vi "MotorControl_PWM+AO.vi"() -> ()   [LabVIEW 2016]
uses:
  <vilib>/Platform/TimedLoop/XDataNode/timing_clust.ctl
  <vilib>/Platform/TimedLoop/XDataNode/nitl_modes.ctl
  <vilib>/Platform/TimedLoop/XDataNode/wakeup.ctl
  <vilib>/rvi/FXPMathLib/FxpDiv/subVIs/nifxpmath_Div_SimConfig.ctl
  <vilib>/rvi/Emulation/niFpgaGetClockAttributes.vi
  <vilib>/rvi/Emulation/niFpgaSctlEmulationGetInTimedLoop.vi
  <vilib>/rvi/Emulation/niFpgaEmulationReportErrorSimple.vi
  <vilib>/rvi/FXPMathLib/FxpDiv/simVIs/DllFxpDivTemp_sub.vi
  GVEncoder.vi
  <vilib>/rvi/Emulation/niFpgaCriticalErrorInLSC.vi
  <vilib>/rvi/Emulation/niFpgaProcessEmulError.vi
  <vilib>/rvi/eio/common/nirviEmuTemplateMethod_errors.vi
  <vilib>/rvi/FXPMathLib/FxpMul/XNode/nifxpmath_Multiplier.xnode
  <vilib>/rvi/FXPMathLib/FxpDiv/XNode/nifxpmath_Div.xnode
  <vilib>/eio/EIONode/EIONode.xnode
  <vilib>/Platform/TimedLoop/XDataNode/XDataNode.xnode
  <vilib>/Platform/TimedLoop/XDataNode/XDNodeRunTimeDep.lvlib
  <vilib>/rvi/FXPMathLib/sim/FxpSim.dll
panel:
  out "ES_PRESSED":bool
  out "PWR_OK":bool
  in  "PWM (Hz/A)":fxp<+/-,32,16>=13.333328247070312 format="%#_21g"
  in  "EncdRst":bool[](array[boolean])=[FALSE, FALSE, FALSE, FALSE, FALSE, FALSE, FALSE, FALSE]
  out "PWM":fxp<+,16,8>[](array[numeric])
  in  "AmpCmd":sgl[](array[numeric])=[0.0, 0.0, 0.0, 0.0, 0.0, 0.0, 0.0, 0.0] format="%#.3f"
  in  "DisableWhenNotReady":bool
  in  "EnableMaster":bool
  out "Ready":bool[](array[boolean])
  in  "Enable":bool[](array[boolean])=[FALSE, FALSE, FALSE, FALSE, FALSE, FALSE, FALSE, FALSE]
  in  "EncoderCount":fxp<+,16,16>=500.0
  in  "2pi":fxp<+/-,32,10>=6.283185243606567 format="%#_39g"
  out "EncdAngle":sgl[](array[numeric]) format="%#.3f"
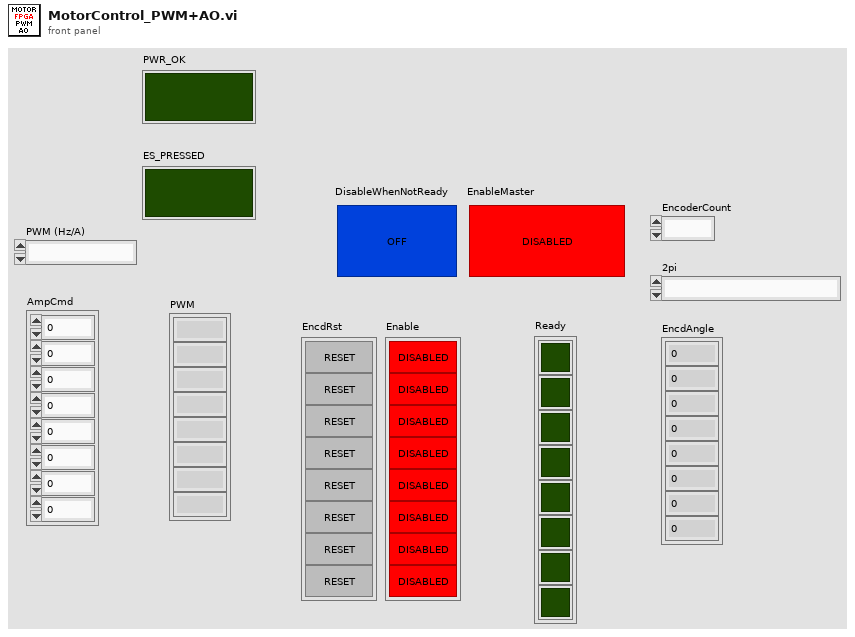
[diagram p1: front panel]
types:
  T1 = typedef "XDNodeRunTimeDep.lvlib/timing_clust.ctl" = cluster{"Expected End [f-1]":u64, "Actual End [f-1]":u64, "Finished Late? [f-1]":bool, "Expected End [i-1]":u64, "Actual End [i-1]":u64, "Finished Late? [i-1]":bool, "Expected Start [i]":u64, "Actual Start [i]":u64, "Expected Start [f]":u64, "Actual Start [f]":u64, "Source Name":string, "Structure Name":string, "Period":i64, "Deadline":i64, "Offset":i64, "Start":i64, "Priority":i32, "Timeout":i32, "Mode":T2, "Wakeup Reason":T3, "Error":errorcluster, "Source Type":string, "Secondary Source Type":string, "Global End Time":u64, "Global Start Time":u64, "Frame Duration":u64, "Iteration Duration":u64, "Assigned CPU":i32, "I/O Scan Engine Mode":u32}
  T2 = typedef "XDNodeRunTimeDep.lvlib/nitl_modes.ctl" = enum32{"No Change", "Process missed periods, maintain original phase", "Discard missed periods, maintain original phase", "Process missed periods, ignore original phase", "Discard missed periods, ignore original phase"}
  T3 = typedef "XDNodeRunTimeDep.lvlib/wakeup.ctl" = enum32{"Normal", "Aborted", "Asynchronous wakeup", "Timing source error", "Timed loop error", "Timeout"}
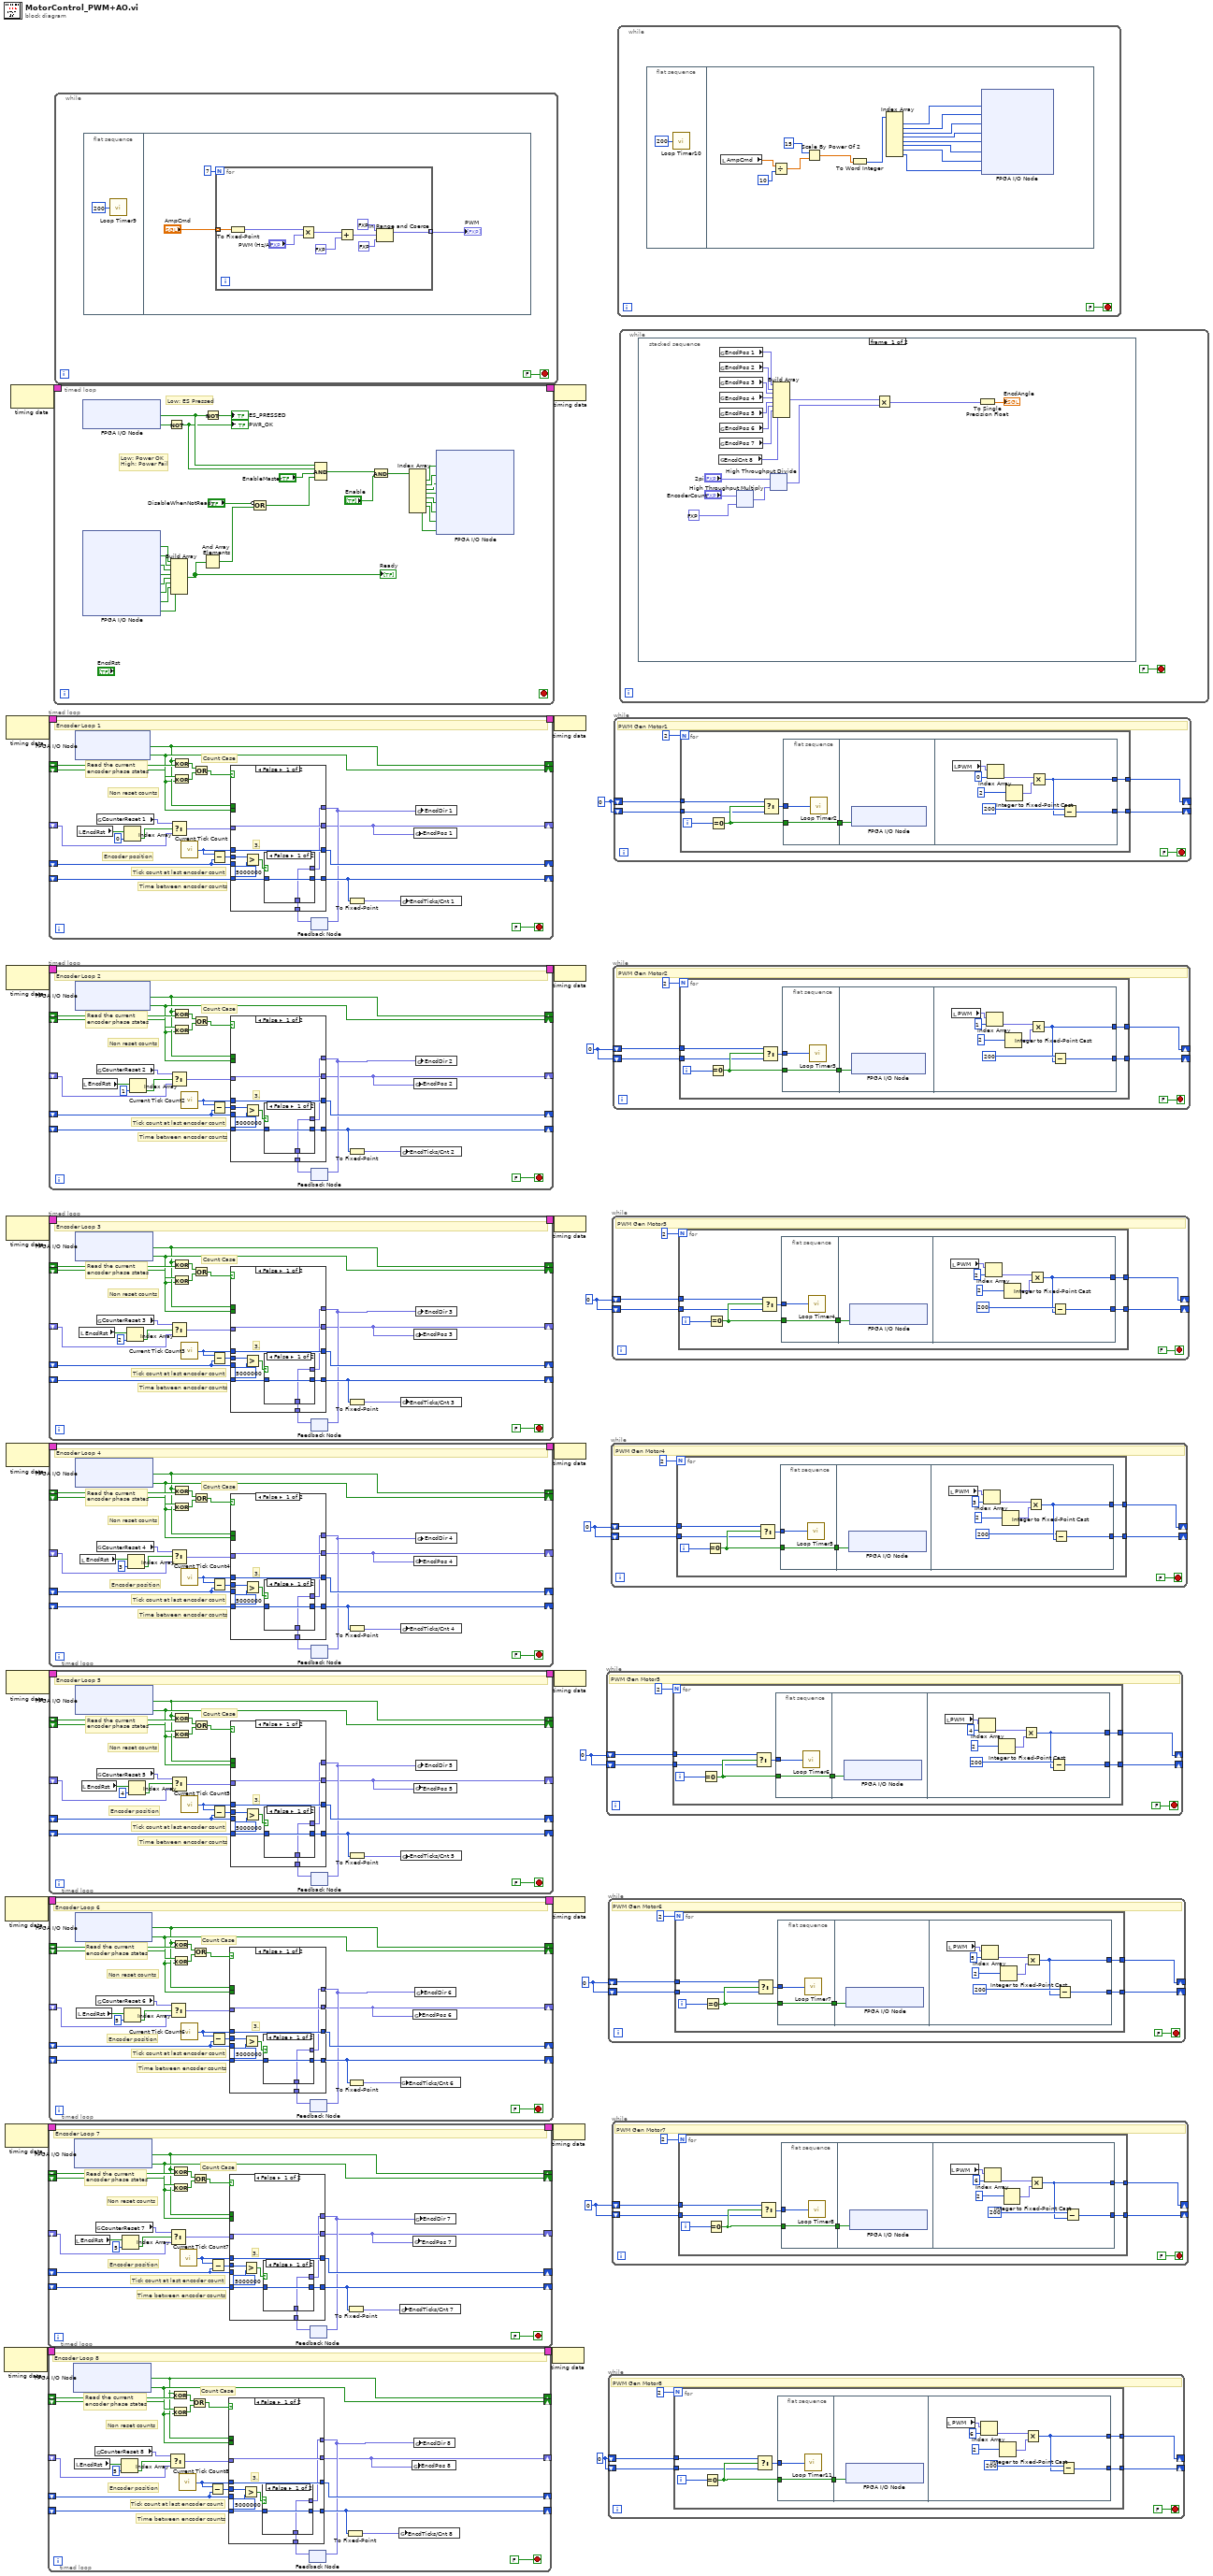
[diagram p0: block diagram]
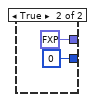
[diagram p2: hidden frame]
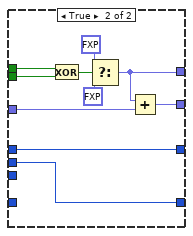
[diagram p3: hidden frame]
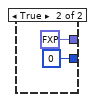
[diagram p4: hidden frame]
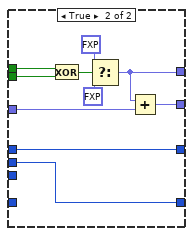
[diagram p5: hidden frame]
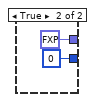
[diagram p6: hidden frame]
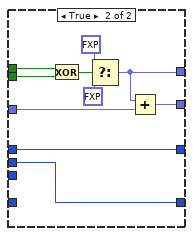
[diagram p7: hidden frame]
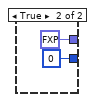
[diagram p8: hidden frame]
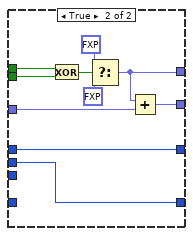
[diagram p9: hidden frame]
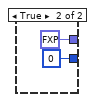
[diagram p10: hidden frame]
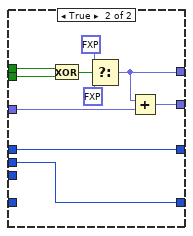
[diagram p11: hidden frame]
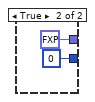
[diagram p12: hidden frame]
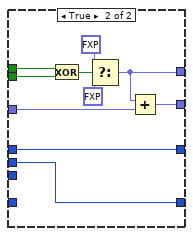
[diagram p13: hidden frame]
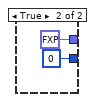
[diagram p14: hidden frame]
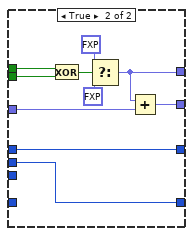
[diagram p15: hidden frame]
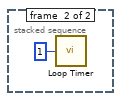
[diagram p16: hidden frame]
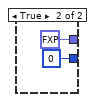
[diagram p17: hidden frame]
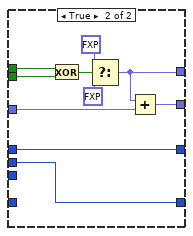
[diagram p18: hidden frame]
diagram:
  w1 = u32 0
  w4 = u32 0
  w5 = u32 0
  w6 = u32 0
  w7 = u32 0
  w8 = u32 0
  w9 = u32 0
  w10 = u32 0
  n1 = node-c288() -> (w3:T1)  [unwired: 1 in]
  n2 = node-c288() -> (w14:T1)  [unwired: 1 in]
  n3 = node-c288() -> (w16:T1)  [unwired: 1 in]
  n4 = node-c288() -> (w26:T1)  [unwired: 1 in]
  n5 = node-c288() -> (w24:T1)  [unwired: 1 in]
  n6 = node-c288() -> (w22:T1)  [unwired: 1 in]
  n7 = node-c288() -> (w20:T1)  [unwired: 1 in]
  n8 = node-c288() -> (w18:T1)  [unwired: 1 in]
  n9 = node-c288() -> (w12:T1)  [unwired: 1 in]
  n10 = timed-loop {
    shift-right: [w44] -> _
    shift-left: _ -> [w50]
    shift-right: [w45] -> _
    shift-left: _ -> [w43]
    shift-right: [w31] -> _
    shift-left: _ -> [w49]
    shift-right: [w48] -> _
    shift-left: _ -> [w42]
    shift-right: [w35] -> _
    shift-left: _ -> [w47]
    timing: w3 -> [_]
    timing-out: [_] -> w2
    stop <- FALSE stop-if-true
    # "Count Case"
    # "Read the current\nencoder phase states"
    # "Non reset counts"
    # "Encoder position"
    # "Time between encoder counts"
    # "Tick count at last encoder count"
    # "Encoder Loop 8"
    n11 = xnode "FPGA I/O Node"() -> ("Connector1/DIO38"=w44:bool, "Connector1/DIO39"=w45:bool)  [unwired: 2 in, 2 out]
    n12 = local read "EncdRst"() -> (w29:bool[])
    n13 = global read "GVEncoder.vi" "CounterReset 8"() -> (w32:fxp<+/-,32,32>)
    n14 = Index Array(array=w29, index=5) -> (element=w27:bool)
    n15 = Select(t=w32, s=w27, f=w49) -> (s? t:f=w38:fxp<+/-,32,32>)
    n16 = Exclusive Or(1:w50, 2:w44) -> (0:w41:bool)
    n17 = Exclusive Or(1:w43, 2:w45) -> (0:w40:bool)
    n18 = call "Current Tick Count8"() -> ("Tick Count(Ticks)"=w36:u32)
    n19 = Or(x=w41, y=w40) -> (x .or. y?=w39:bool)
    n20 = Subtract(x=w36, y=w42) -> (x-y=w37:u32)
    n21 = feedback #1() -> (w34:fxp<+/-,2,2>)  [unwired: 1 in]
    n22 = case shown="False" w39 {
      tunnel: [w59 w67] -> w31
      tunnel: w38 -> [w59 w73]
      tunnel: [w53 w66] -> w48
      tunnel: w42 -> [w53 _]
      tunnel: [w56 w65] -> w35
      tunnel: w47 -> [w55 _]
      tunnel: w44 -> [_ w69]
      tunnel: w43 -> [_ w68]
      tunnel: w37 -> [w54 w65]
      tunnel: w36 -> [_ w66]
      tunnel: [w52 w64] -> w33
      tunnel: w34 -> [w51 _]
      frame False {
        # "3."
        n23 = Greater?(x=w54, y=u32 5000000 ("x")) -> (0:w57:bool)
        n24 = case shown="False" w57 {
          tunnel: [w61 u32 0 ("x")] -> w56
          tunnel: w55 -> [w61 _]
          tunnel: [w60 fxp<+/-,2,2> 0.0 ("16 bit")] -> w52
          tunnel: w51 -> [w60 _]
          frame False {
          }
          frame True {
          }
        }
      }
      frame True {
        n25 = Exclusive Or(1:w68, 2:w69) -> (0:w70:bool)
        n26 = Select(t=fxp<+,1,1> 1.0 ("16 bit"), s=w70, f=fxp<+/-,1,1> -1.0 ("16 bit")) -> (s? t:f=w64:fxp<+/-,2,2>)
        n27 = Add(x=w64, y=w73) -> (x+y=w67:fxp<+/-,32,32>)
      }
    }
    n28 = feedback-in #1(w33) -> ()
    n29 = To Fixed-Point(number=w35) -> (fixed-point=w30:fxp<+,32,32>)  [unwired: 1 in]
    n30 = global write "GVEncoder.vi" "EncdTicks/Cnt 8"(w30) -> ()
    n31 = global write "GVEncoder.vi" "EncdPos 8"(w31) -> ()
    n32 = global write "GVEncoder.vi" "EncdDir 8"(w33) -> ()
  }
  n33 = timed-loop {
    shift-right: [w93] -> _
    shift-left: _ -> [w99]
    shift-right: [w94] -> _
    shift-left: _ -> [w92]
    shift-right: [w80] -> _
    shift-left: _ -> [w98]
    shift-right: [w97] -> _
    shift-left: _ -> [w91]
    shift-right: [w84] -> _
    shift-left: _ -> [w96]
    timing: w14 -> [_]
    timing-out: [_] -> w13
    stop <- FALSE stop-if-true
    # "Count Case"
    # "Read the current\nencoder phase states"
    # "Non reset counts"
    # "Encoder position"
    # "Time between encoder counts"
    # "Tick count at last encoder count"
    # "Encoder Loop 7"
    n34 = xnode "FPGA I/O Node"() -> ("Connector1/DIO33"=w93:bool, "Connector1/DIO34"=w94:bool)  [unwired: 2 in, 2 out]
    n35 = local read "EncdRst"() -> (w78:bool[])
    n36 = global read "GVEncoder.vi" "CounterReset 7"() -> (w81:fxp<+/-,32,32>)
    n37 = Index Array(array=w78, index=5) -> (element=w76:bool)
    n38 = Select(t=w81, s=w76, f=w98) -> (s? t:f=w87:fxp<+/-,32,32>)
    n39 = Exclusive Or(1:w99, 2:w93) -> (0:w90:bool)
    n40 = Exclusive Or(1:w92, 2:w94) -> (0:w89:bool)
    n41 = call "Current Tick Count7"() -> ("Tick Count(Ticks)"=w85:u32)
    n42 = Or(x=w90, y=w89) -> (x .or. y?=w88:bool)
    n43 = Subtract(x=w85, y=w91) -> (x-y=w86:u32)
    n44 = feedback #2() -> (w83:fxp<+/-,2,2>)  [unwired: 1 in]
    n45 = case shown="False" w88 {
      tunnel: [w108 w116] -> w80
      tunnel: w87 -> [w108 w122]
      tunnel: [w102 w115] -> w97
      tunnel: w91 -> [w102 _]
      tunnel: [w105 w114] -> w84
      tunnel: w96 -> [w104 _]
      tunnel: w93 -> [_ w118]
      tunnel: w92 -> [_ w117]
      tunnel: w86 -> [w103 w114]
      tunnel: w85 -> [_ w115]
      tunnel: [w101 w113] -> w82
      tunnel: w83 -> [w100 _]
      frame False {
        # "3."
        n46 = Greater?(x=w103, y=u32 5000000 ("x")) -> (0:w106:bool)
        n47 = case shown="False" w106 {
          tunnel: [w110 u32 0 ("x")] -> w105
          tunnel: w104 -> [w110 _]
          tunnel: [w109 fxp<+/-,2,2> 0.0 ("16 bit")] -> w101
          tunnel: w100 -> [w109 _]
          frame False {
          }
          frame True {
          }
        }
      }
      frame True {
        n48 = Exclusive Or(1:w117, 2:w118) -> (0:w119:bool)
        n49 = Select(t=fxp<+,1,1> 1.0 ("16 bit"), s=w119, f=fxp<+/-,1,1> -1.0 ("16 bit")) -> (s? t:f=w113:fxp<+/-,2,2>)
        n50 = Add(x=w113, y=w122) -> (x+y=w116:fxp<+/-,32,32>)
      }
    }
    n51 = feedback-in #2(w82) -> ()
    n52 = To Fixed-Point(number=w84) -> (fixed-point=w79:fxp<+,32,32>)  [unwired: 1 in]
    n53 = global write "GVEncoder.vi" "EncdTicks/Cnt 7"(w79) -> ()
    n54 = global write "GVEncoder.vi" "EncdPos 7"(w80) -> ()
    n55 = global write "GVEncoder.vi" "EncdDir 7"(w82) -> ()
  }
  n56 = timed-loop {
    shift-right: [w142] -> _
    shift-left: _ -> [w148]
    shift-right: [w143] -> _
    shift-left: _ -> [w141]
    shift-right: [w129] -> _
    shift-left: _ -> [w147]
    shift-right: [w146] -> _
    shift-left: _ -> [w140]
    shift-right: [w133] -> _
    shift-left: _ -> [w145]
    timing: w16 -> [_]
    timing-out: [_] -> w15
    stop <- FALSE stop-if-true
    # "Count Case"
    # "Read the current\nencoder phase states"
    # "Non reset counts"
    # "Encoder position"
    # "Time between encoder counts"
    # "Tick count at last encoder count"
    # "Encoder Loop 6"
    n57 = xnode "FPGA I/O Node"() -> ("Connector1/DIO28"=w142:bool, "Connector1/DIO29"=w143:bool)  [unwired: 2 in, 2 out]
    n58 = local read "EncdRst"() -> (w126:bool[])
    n59 = global read "GVEncoder.vi" "CounterReset 6"() -> (w130:fxp<+/-,32,32>)
    n60 = Index Array(array=w126, index=5) -> (element=w125:bool)
    n61 = Select(t=w130, s=w125, f=w147) -> (s? t:f=w136:fxp<+/-,32,32>)
    n62 = Exclusive Or(1:w148, 2:w142) -> (0:w139:bool)
    n63 = Exclusive Or(1:w141, 2:w143) -> (0:w138:bool)
    n64 = call "Current Tick Count6"() -> ("Tick Count(Ticks)"=w134:u32)
    n65 = Or(x=w139, y=w138) -> (x .or. y?=w137:bool)
    n66 = Subtract(x=w134, y=w140) -> (x-y=w135:u32)
    n67 = feedback #3() -> (w132:fxp<+/-,2,2>)  [unwired: 1 in]
    n68 = case shown="False" w137 {
      tunnel: [w157 w165] -> w129
      tunnel: w136 -> [w157 w171]
      tunnel: [w151 w164] -> w146
      tunnel: w140 -> [w151 _]
      tunnel: [w154 w163] -> w133
      tunnel: w145 -> [w153 _]
      tunnel: w142 -> [_ w167]
      tunnel: w141 -> [_ w166]
      tunnel: w135 -> [w152 w163]
      tunnel: w134 -> [_ w164]
      tunnel: [w150 w162] -> w131
      tunnel: w132 -> [w149 _]
      frame False {
        # "3."
        n69 = Greater?(x=w152, y=u32 5000000 ("x")) -> (0:w155:bool)
        n70 = case shown="False" w155 {
          tunnel: [w159 u32 0 ("x")] -> w154
          tunnel: w153 -> [w159 _]
          tunnel: [w158 fxp<+/-,2,2> 0.0 ("16 bit")] -> w150
          tunnel: w149 -> [w158 _]
          frame False {
          }
          frame True {
          }
        }
      }
      frame True {
        n71 = Exclusive Or(1:w166, 2:w167) -> (0:w168:bool)
        n72 = Select(t=fxp<+,1,1> 1.0 ("16 bit"), s=w168, f=fxp<+/-,1,1> -1.0 ("16 bit")) -> (s? t:f=w162:fxp<+/-,2,2>)
        n73 = Add(x=w162, y=w171) -> (x+y=w165:fxp<+/-,32,32>)
      }
    }
    n74 = feedback-in #3(w131) -> ()
    n75 = To Fixed-Point(number=w133) -> (fixed-point=w128:fxp<+,32,32>)  [unwired: 1 in]
    n76 = global write "GVEncoder.vi" "EncdTicks/Cnt 6"(w128) -> ()
    n77 = global write "GVEncoder.vi" "EncdPos 6"(w129) -> ()
    n78 = global write "GVEncoder.vi" "EncdDir 6"(w131) -> ()
  }
  n79 = timed-loop {
    shift-right: [w191] -> _
    shift-left: _ -> [w197]
    shift-right: [w192] -> _
    shift-left: _ -> [w190]
    shift-right: [w178] -> _
    shift-left: _ -> [w196]
    shift-right: [w195] -> _
    shift-left: _ -> [w189]
    shift-right: [w182] -> _
    shift-left: _ -> [w194]
    timing: w26 -> [_]
    timing-out: [_] -> w25
    stop <- FALSE stop-if-true
    # "Count Case"
    # "Read the current\nencoder phase states"
    # "Non reset counts"
    # "Encoder position"
    # "Time between encoder counts"
    # "Tick count at last encoder count"
    # "Encoder Loop 1"
    n80 = xnode "FPGA I/O Node"() -> ("Connector1/DIO3"=w191:bool, "Connector1/DIO4"=w192:bool)  [unwired: 2 in, 2 out]
    n81 = local read "EncdRst"() -> (w176:bool[])
    n82 = global read "GVEncoder.vi" "CounterReset 1"() -> (w179:fxp<+/-,32,32>)
    n83 = Index Array(array=w176, index=0) -> (element=w174:bool)
    n84 = Select(t=w179, s=w174, f=w196) -> (s? t:f=w185:fxp<+/-,32,32>)
    n85 = Exclusive Or(1:w197, 2:w191) -> (0:w188:bool)
    n86 = Exclusive Or(1:w190, 2:w192) -> (0:w187:bool)
    n87 = call "Current Tick Count"() -> ("Tick Count(Ticks)"=w183:u32)
    n88 = Or(x=w188, y=w187) -> (x .or. y?=w186:bool)
    n89 = Subtract(x=w183, y=w189) -> (x-y=w184:u32)
    n90 = feedback #4() -> (w181:fxp<+/-,2,2>)  [unwired: 1 in]
    n91 = case shown="False" w186 {
      tunnel: [w206 w214] -> w178
      tunnel: w185 -> [w206 w220]
      tunnel: [w200 w213] -> w195
      tunnel: w189 -> [w200 _]
      tunnel: [w203 w212] -> w182
      tunnel: w194 -> [w202 _]
      tunnel: w191 -> [_ w216]
      tunnel: w190 -> [_ w215]
      tunnel: w184 -> [w201 w212]
      tunnel: w183 -> [_ w213]
      tunnel: [w199 w211] -> w180
      tunnel: w181 -> [w198 _]
      frame False {
        # "3."
        n92 = Greater?(x=w201, y=u32 5000000 ("x")) -> (0:w204:bool)
        n93 = case shown="False" w204 {
          tunnel: [w208 u32 0 ("x")] -> w203
          tunnel: w202 -> [w208 _]
          tunnel: [w207 fxp<+/-,2,2> 0.0 ("16 bit")] -> w199
          tunnel: w198 -> [w207 _]
          frame False {
          }
          frame True {
          }
        }
      }
      frame True {
        n94 = Exclusive Or(1:w215, 2:w216) -> (0:w217:bool)
        n95 = Select(t=fxp<+,1,1> 1.0 ("16 bit"), s=w217, f=fxp<+/-,1,1> -1.0 ("16 bit")) -> (s? t:f=w211:fxp<+/-,2,2>)
        n96 = Add(x=w211, y=w220) -> (x+y=w214:fxp<+/-,32,32>)
      }
    }
    n97 = feedback-in #4(w180) -> ()
    n98 = To Fixed-Point(number=w182) -> (fixed-point=w177:fxp<+,32,32>)  [unwired: 1 in]
    n99 = global write "GVEncoder.vi" "EncdTicks/Cnt 1"(w177) -> ()
    n100 = global write "GVEncoder.vi" "EncdPos 1"(w178) -> ()
    n101 = global write "GVEncoder.vi" "EncdDir 1"(w180) -> ()
  }
  n102 = timed-loop {
    shift-right: [w240] -> _
    shift-left: _ -> [w246]
    shift-right: [w241] -> _
    shift-left: _ -> [w239]
    shift-right: [w227] -> _
    shift-left: _ -> [w245]
    shift-right: [w244] -> _
    shift-left: _ -> [w238]
    shift-right: [w231] -> _
    shift-left: _ -> [w243]
    timing: w24 -> [_]
    timing-out: [_] -> w23
    stop <- FALSE stop-if-true
    # "Count Case"
    # "Read the current\nencoder phase states"
    # "Non reset counts"
    # "Time between encoder counts"
    # "Tick count at last encoder count"
    # "Encoder Loop 2"
    n103 = xnode "FPGA I/O Node"() -> ("Connector1/DIO8"=w240:bool, "Connector1/DIO9"=w241:bool)  [unwired: 2 in, 2 out]
    n104 = local read "EncdRst"() -> (w224:bool[])
    n105 = global read "GVEncoder.vi" "CounterReset 2"() -> (w228:fxp<+/-,32,32>)
    n106 = Index Array(array=w224, index=1) -> (element=w223:bool)
    n107 = Select(t=w228, s=w223, f=w245) -> (s? t:f=w234:fxp<+/-,32,32>)
    n108 = Exclusive Or(1:w246, 2:w240) -> (0:w237:bool)
    n109 = Exclusive Or(1:w239, 2:w241) -> (0:w236:bool)
    n110 = call "Current Tick Count2"() -> ("Tick Count(Ticks)"=w232:u32)
    n111 = Or(x=w237, y=w236) -> (x .or. y?=w235:bool)
    n112 = Subtract(x=w232, y=w238) -> (x-y=w233:u32)
    n113 = feedback #5() -> (w230:fxp<+/-,2,2>)  [unwired: 1 in]
    n114 = case shown="False" w235 {
      tunnel: [w255 w263] -> w227
      tunnel: w234 -> [w255 w269]
      tunnel: [w249 w262] -> w244
      tunnel: w238 -> [w249 _]
      tunnel: [w252 w261] -> w231
      tunnel: w243 -> [w251 _]
      tunnel: w240 -> [_ w265]
      tunnel: w239 -> [_ w264]
      tunnel: w233 -> [w250 w261]
      tunnel: w232 -> [_ w262]
      tunnel: [w248 w260] -> w229
      tunnel: w230 -> [w247 _]
      frame False {
        # "3."
        n115 = Greater?(x=w250, y=u32 5000000 ("x")) -> (0:w253:bool)
        n116 = case shown="False" w253 {
          tunnel: [w257 u32 0 ("x")] -> w252
          tunnel: w251 -> [w257 _]
          tunnel: [w256 fxp<+/-,2,2> 0.0 ("16 bit")] -> w248
          tunnel: w247 -> [w256 _]
          frame False {
          }
          frame True {
          }
        }
      }
      frame True {
        n117 = Exclusive Or(1:w264, 2:w265) -> (0:w266:bool)
        n118 = Select(t=fxp<+,1,1> 1.0 ("16 bit"), s=w266, f=fxp<+/-,1,1> -1.0 ("16 bit")) -> (s? t:f=w260:fxp<+/-,2,2>)
        n119 = Add(x=w260, y=w269) -> (x+y=w263:fxp<+/-,32,32>)
      }
    }
    n120 = feedback-in #5(w229) -> ()
    n121 = To Fixed-Point(number=w231) -> (fixed-point=w226:fxp<+,32,32>)  [unwired: 1 in]
    n122 = global write "GVEncoder.vi" "EncdTicks/Cnt 2"(w226) -> ()
    n123 = global write "GVEncoder.vi" "EncdPos 2"(w227) -> ()
    n124 = global write "GVEncoder.vi" "EncdDir 2"(w229) -> ()
  }
  n125 = timed-loop {
    shift-right: [w289] -> _
    shift-left: _ -> [w295]
    shift-right: [w290] -> _
    shift-left: _ -> [w288]
    shift-right: [w276] -> _
    shift-left: _ -> [w294]
    shift-right: [w293] -> _
    shift-left: _ -> [w287]
    shift-right: [w280] -> _
    shift-left: _ -> [w292]
    timing: w22 -> [_]
    timing-out: [_] -> w21
    stop <- FALSE stop-if-true
    # "Count Case"
    # "Read the current\nencoder phase states"
    # "Non reset counts"
    # "Time between encoder counts"
    # "Tick count at last encoder count"
    # "Encoder Loop 3"
    n126 = xnode "FPGA I/O Node"() -> ("Connector1/DIO13"=w289:bool, "Connector1/DIO14"=w290:bool)  [unwired: 2 in, 2 out]
    n127 = local read "EncdRst"() -> (w274:bool[])
    n128 = global read "GVEncoder.vi" "CounterReset 3"() -> (w277:fxp<+/-,32,32>)
    n129 = Index Array(array=w274, index=2) -> (element=w272:bool)
    n130 = Select(t=w277, s=w272, f=w294) -> (s? t:f=w283:fxp<+/-,32,32>)
    n131 = Exclusive Or(1:w295, 2:w289) -> (0:w286:bool)
    n132 = Exclusive Or(1:w288, 2:w290) -> (0:w285:bool)
    n133 = call "Current Tick Count3"() -> ("Tick Count(Ticks)"=w281:u32)
    n134 = Or(x=w286, y=w285) -> (x .or. y?=w284:bool)
    n135 = Subtract(x=w281, y=w287) -> (x-y=w282:u32)
    n136 = feedback #6() -> (w279:fxp<+/-,2,2>)  [unwired: 1 in]
    n137 = case shown="False" w284 {
      tunnel: [w304 w312] -> w276
      tunnel: w283 -> [w304 w318]
      tunnel: [w298 w311] -> w293
      tunnel: w287 -> [w298 _]
      tunnel: [w301 w310] -> w280
      tunnel: w292 -> [w300 _]
      tunnel: w289 -> [_ w314]
      tunnel: w288 -> [_ w313]
      tunnel: w282 -> [w299 w310]
      tunnel: w281 -> [_ w311]
      tunnel: [w297 w309] -> w278
      tunnel: w279 -> [w296 _]
      frame False {
        # "3."
        n138 = Greater?(x=w299, y=u32 5000000 ("x")) -> (0:w302:bool)
        n139 = case shown="False" w302 {
          tunnel: [w306 u32 0 ("x")] -> w301
          tunnel: w300 -> [w306 _]
          tunnel: [w305 fxp<+/-,2,2> 0.0 ("16 bit")] -> w297
          tunnel: w296 -> [w305 _]
          frame False {
          }
          frame True {
          }
        }
      }
      frame True {
        n140 = Exclusive Or(1:w313, 2:w314) -> (0:w315:bool)
        n141 = Select(t=fxp<+,1,1> 1.0 ("16 bit"), s=w315, f=fxp<+/-,1,1> -1.0 ("16 bit")) -> (s? t:f=w309:fxp<+/-,2,2>)
        n142 = Add(x=w309, y=w318) -> (x+y=w312:fxp<+/-,32,32>)
      }
    }
    n143 = feedback-in #6(w278) -> ()
    n144 = To Fixed-Point(number=w280) -> (fixed-point=w275:fxp<+,32,32>)  [unwired: 1 in]
    n145 = global write "GVEncoder.vi" "EncdTicks/Cnt 3"(w275) -> ()
    n146 = global write "GVEncoder.vi" "EncdPos 3"(w276) -> ()
    n147 = global write "GVEncoder.vi" "EncdDir 3"(w278) -> ()
  }
  n148 = timed-loop {
    shift-right: [w338] -> _
    shift-left: _ -> [w344]
    shift-right: [w339] -> _
    shift-left: _ -> [w337]
    shift-right: [w325] -> _
    shift-left: _ -> [w343]
    shift-right: [w342] -> _
    shift-left: _ -> [w336]
    shift-right: [w329] -> _
    shift-left: _ -> [w341]
    timing: w20 -> [_]
    timing-out: [_] -> w19
    stop <- FALSE stop-if-true
    # "Count Case"
    # "Read the current\nencoder phase states"
    # "Non reset counts"
    # "Encoder position"
    # "Time between encoder counts"
    # "Tick count at last encoder count"
    # "Encoder Loop 4"
    n149 = xnode "FPGA I/O Node"() -> ("Connector1/DIO18"=w338:bool, "Connector1/DIO19"=w339:bool)  [unwired: 2 in, 2 out]
    n150 = local read "EncdRst"() -> (w322:bool[])
    n151 = global read "GVEncoder.vi" "CounterReset 4"() -> (w326:fxp<+/-,32,32>)
    n152 = Index Array(array=w322, index=3) -> (element=w321:bool)
    n153 = Select(t=w326, s=w321, f=w343) -> (s? t:f=w332:fxp<+/-,32,32>)
    n154 = Exclusive Or(1:w344, 2:w338) -> (0:w335:bool)
    n155 = Exclusive Or(1:w337, 2:w339) -> (0:w334:bool)
    n156 = call "Current Tick Count4"() -> ("Tick Count(Ticks)"=w330:u32)
    n157 = Or(x=w335, y=w334) -> (x .or. y?=w333:bool)
    n158 = Subtract(x=w330, y=w336) -> (x-y=w331:u32)
    n159 = feedback #7() -> (w328:fxp<+/-,2,2>)  [unwired: 1 in]
    n160 = case shown="False" w333 {
      tunnel: [w353 w361] -> w325
      tunnel: w332 -> [w353 w367]
      tunnel: [w347 w360] -> w342
      tunnel: w336 -> [w347 _]
      tunnel: [w350 w359] -> w329
      tunnel: w341 -> [w349 _]
      tunnel: w338 -> [_ w363]
      tunnel: w337 -> [_ w362]
      tunnel: w331 -> [w348 w359]
      tunnel: w330 -> [_ w360]
      tunnel: [w346 w358] -> w327
      tunnel: w328 -> [w345 _]
      frame False {
        # "3."
        n161 = Greater?(x=w348, y=u32 5000000 ("x")) -> (0:w351:bool)
        n162 = case shown="False" w351 {
          tunnel: [w355 u32 0 ("x")] -> w350
          tunnel: w349 -> [w355 _]
          tunnel: [w354 fxp<+/-,2,2> 0.0 ("16 bit")] -> w346
          tunnel: w345 -> [w354 _]
          frame False {
          }
          frame True {
          }
        }
      }
      frame True {
        n163 = Exclusive Or(1:w362, 2:w363) -> (0:w364:bool)
        n164 = Select(t=fxp<+,1,1> 1.0 ("16 bit"), s=w364, f=fxp<+/-,1,1> -1.0 ("16 bit")) -> (s? t:f=w358:fxp<+/-,2,2>)
        n165 = Add(x=w358, y=w367) -> (x+y=w361:fxp<+/-,32,32>)
      }
    }
    n166 = feedback-in #7(w327) -> ()
    n167 = To Fixed-Point(number=w329) -> (fixed-point=w324:fxp<+,32,32>)  [unwired: 1 in]
    n168 = global write "GVEncoder.vi" "EncdTicks/Cnt 4"(w324) -> ()
    n169 = global write "GVEncoder.vi" "EncdPos 4"(w325) -> ()
    n170 = global write "GVEncoder.vi" "EncdDir 4"(w327) -> ()
  }
  n171 = timed-loop {
    shift-right: [w387] -> _
    shift-left: _ -> [w393]
    shift-right: [w388] -> _
    shift-left: _ -> [w386]
    shift-right: [w374] -> _
    shift-left: _ -> [w392]
    shift-right: [w391] -> _
    shift-left: _ -> [w385]
    shift-right: [w378] -> _
    shift-left: _ -> [w390]
    timing: w18 -> [_]
    timing-out: [_] -> w17
    stop <- FALSE stop-if-true
    # "Count Case"
    # "Read the current\nencoder phase states"
    # "Non reset counts"
    # "Encoder position"
    # "Time between encoder counts"
    # "Tick count at last encoder count"
    # "Encoder Loop 5"
    n172 = xnode "FPGA I/O Node"() -> ("Connector1/DIO23"=w387:bool, "Connector1/DIO24"=w388:bool)  [unwired: 2 in, 2 out]
    n173 = local read "EncdRst"() -> (w372:bool[])
    n174 = global read "GVEncoder.vi" "CounterReset 5"() -> (w375:fxp<+/-,32,32>)
    n175 = Index Array(array=w372, index=4) -> (element=w370:bool)
    n176 = Select(t=w375, s=w370, f=w392) -> (s? t:f=w381:fxp<+/-,32,32>)
    n177 = Exclusive Or(1:w393, 2:w387) -> (0:w384:bool)
    n178 = Exclusive Or(1:w386, 2:w388) -> (0:w383:bool)
    n179 = call "Current Tick Count5"() -> ("Tick Count(Ticks)"=w379:u32)
    n180 = Or(x=w384, y=w383) -> (x .or. y?=w382:bool)
    n181 = Subtract(x=w379, y=w385) -> (x-y=w380:u32)
    n182 = feedback #8() -> (w377:fxp<+/-,2,2>)  [unwired: 1 in]
    n183 = case shown="False" w382 {
      tunnel: [w402 w410] -> w374
      tunnel: w381 -> [w402 w416]
      tunnel: [w396 w409] -> w391
      tunnel: w385 -> [w396 _]
      tunnel: [w399 w408] -> w378
      tunnel: w390 -> [w398 _]
      tunnel: w387 -> [_ w412]
      tunnel: w386 -> [_ w411]
      tunnel: w380 -> [w397 w408]
      tunnel: w379 -> [_ w409]
      tunnel: [w395 w407] -> w376
      tunnel: w377 -> [w394 _]
      frame False {
        # "3."
        n184 = Greater?(x=w397, y=u32 5000000 ("x")) -> (0:w400:bool)
        n185 = case shown="False" w400 {
          tunnel: [w404 u32 0 ("x")] -> w399
          tunnel: w398 -> [w404 _]
          tunnel: [w403 fxp<+/-,2,2> 0.0 ("16 bit")] -> w395
          tunnel: w394 -> [w403 _]
          frame False {
          }
          frame True {
          }
        }
      }
      frame True {
        n186 = Exclusive Or(1:w411, 2:w412) -> (0:w413:bool)
        n187 = Select(t=fxp<+,1,1> 1.0 ("16 bit"), s=w413, f=fxp<+/-,1,1> -1.0 ("16 bit")) -> (s? t:f=w407:fxp<+/-,2,2>)
        n188 = Add(x=w407, y=w416) -> (x+y=w410:fxp<+/-,32,32>)
      }
    }
    n189 = feedback-in #8(w376) -> ()
    n190 = To Fixed-Point(number=w378) -> (fixed-point=w373:fxp<+,32,32>)  [unwired: 1 in]
    n191 = global write "GVEncoder.vi" "EncdTicks/Cnt 5"(w373) -> ()
    n192 = global write "GVEncoder.vi" "EncdPos 5"(w374) -> ()
    n193 = global write "GVEncoder.vi" "EncdDir 5"(w376) -> ()
  }
  n194 = timed-loop {
    timing: w12 -> [_]
    timing-out: [_] -> w11
    stop <- _ stop-if-true
    # "Low: ES Pressed"
    # "Low: Power OK\nHigh: Power Fail"
    n195 = xnode "FPGA I/O Node"() -> ("Connector1/DIO37"=w425:bool, "Connector1/DIO36"=w424:bool)  [unwired: 2 in, 2 out]
    n196 = xnode "FPGA I/O Node"() -> ("Connector1/DIO2"=w444:bool, "Connector1/DIO7"=w443:bool, "Connector1/DIO12"=w442:bool, "Connector1/DIO17"=w441:bool, "Connector1/DIO22"=w440:bool, "Connector1/DIO27"=w439:bool, "Connector1/DIO32"=w438:bool, "Connector1/DIO37"=w420:bool)  [unwired: 8 in, 8 out]
    n197 = Not(x=w424) -> (.not. x?=w422:bool)
    "PWR_OK" <- w422
    n198 = Build Array(w444, w443, w442, w441, w440, w439, w438, w420) -> (w421:bool[])
    "Ready" <- w421
    n199 = And Array Elements(Boolean array=w421) -> (logical AND=w436:bool)
    n200 = Not(x=w425) -> (.not. x?=→"ES_PRESSED":bool)
    n201 = Compound Arithmetic op=OR(invert "DisableWhenNotReady", w436) -> (w427:bool)
    n202 = Compound Arithmetic op=AND(w425, w422, "EnableMaster", w427) -> (w428:bool)
    n203 = And(x=w428, y="Enable") -> (x .and. y?=w445:bool[])
    n204 = Index Array(array=w445) -> (element #1=w435:bool, element #2=w434:bool, element #3=w433:bool, element #4=w432:bool, element #5=w431:bool, element #6=w430:bool, element #7=w429:bool, element #8=w419:bool)  [unwired: 8 in]
    n205 = xnode "FPGA I/O Node"("Connector1/DIO1"=w435, "Connector1/DIO6"=w434, "Connector1/DIO11"=w433, "Connector1/DIO16"=w432, "Connector1/DIO21"=w431, "Connector1/DIO26"=w430, "Connector1/DIO31"=w429, "Connector1/DIO36"=w419) -> ()  [unwired: 8 in, 8 out]
  }
  n206 = while {
    stop <- FALSE stop-if-true
    n207 = flat-sequence {
      frame #0 {
        n208 = call "Loop Timer9"("Count(uSec)"=u32 200) -> ()  [unwired: 1 out]
      }
      frame #1 {
        n209 = for {
          N: 7 -> [_]
          tunnel: "AmpCmd" -> [w462] mode=indexing
          tunnel: [w454] -> w451 mode=indexing
          n210 = To Fixed-Point(number=w462) -> (fixed-point=w461:fxp<+/-,32,16>)  [unwired: 1 in]
          n211 = Multiply(x=w461, y="PWM (Hz/A)") -> (x*y=w459:fxp<+/-,16,8>)
          n212 = Add(x=w459, y=fxp<+,16,8> 50.0) -> (x+y=w455:fxp<+,16,8>)
          n213 = In Range and Coerce(upper limit=fxp<+,16,8> 90.0 ("y"), x=w455, lower limit=fxp<+,16,8> 10.0 ("y")) -> (coerced(x)=w454:fxp<+,16,8>)  [unwired: 1 out]
        }
        "PWM" <- w451
      }
    }
  }
  n214 = node-c288(w2) -> ()
  n215 = node-c288(w13) -> ()
  n216 = node-c288(w15) -> ()
  n217 = node-c288(w25) -> ()
  n218 = node-c288(w23) -> ()
  n219 = node-c288(w21) -> ()
  n220 = node-c288(w19) -> ()
  n221 = node-c288(w17) -> ()
  n222 = node-c288(w11) -> ()
  n223 = while {
    shift-right: [w464] -> _
    shift-left: w7 -> [w467]
    shift-right: [w465] -> _
    shift-left: w7 -> [w466]
    stop <- FALSE stop-if-true
    # "PWM Gen Motor5"
    n224 = for {
      N: 2 -> [_]
      tunnel: w467 -> [w471]
      tunnel: w466 -> [w472]
      tunnel: [w470] -> w465
      tunnel: [w469] -> w464
      i -> [w476]
      n225 = Equal To 0?(x=w476) -> (x = 0?=w473:bool)
      n226 = Select(t=w471, s=w473, f=w472) -> (s? t:f=w475:u32)
      n227 = flat-sequence {
        tunnel: w475 -> [w477]
        tunnel: [w478] -> w474
        tunnel: w473 -> [w478]
        tunnel: w474 -> [w479]
        tunnel: [w487] -> w470
        tunnel: [w480] -> w469
        frame #0 {
          n228 = call "Loop Timer6"("Count(uSec)"=w477) -> ()  [unwired: 1 out]
        }
        frame #1 {
          n229 = xnode "FPGA I/O Node"("Connector1/DIO20"=w479) -> ()  [unwired: 1 in, 1 out]
        }
        frame #2 {
          n230 = local read "PWM"() -> (w484:fxp<+,16,8>[])
          n231 = Index Array(array=w484, index=4) -> (element=w483:fxp<+,16,8>)
          n232 = Integer to Fixed-Point Cast(integer=u32 2) -> (fixed-point=w485:fxp<+,32,32>)  [unwired: 1 in]
          n233 = Multiply(x=w483, y=w485) -> (x*y=w480:u32)
          n234 = Subtract(x=u32 200, y=w480) -> (x-y=w487:u32)
        }
      }
    }
  }
  n235 = while {
    shift-right: [w489] -> _
    shift-left: w1 -> [w492]
    shift-right: [w490] -> _
    shift-left: w1 -> [w491]
    stop <- FALSE stop-if-true
    # "PWM Gen Motor8"
    n236 = for {
      N: 2 -> [_]
      tunnel: w492 -> [w496]
      tunnel: w491 -> [w497]
      tunnel: [w495] -> w490
      tunnel: [w494] -> w489
      i -> [w501]
      n237 = Equal To 0?(x=w501) -> (x = 0?=w498:bool)
      n238 = Select(t=w496, s=w498, f=w497) -> (s? t:f=w500:u32)
      n239 = flat-sequence {
        tunnel: w500 -> [w502]
        tunnel: [w503] -> w499
        tunnel: w498 -> [w503]
        tunnel: w499 -> [w504]
        tunnel: [w512] -> w495
        tunnel: [w505] -> w494
        frame #0 {
          n240 = call "Loop Timer11"("Count(uSec)"=w502) -> ()  [unwired: 1 out]
        }
        frame #1 {
          n241 = xnode "FPGA I/O Node"("Connector1/DIO35"=w504) -> ()  [unwired: 1 in, 1 out]
        }
        frame #2 {
          n242 = local read "PWM"() -> (w509:fxp<+,16,8>[])
          n243 = Index Array(array=w509, index=6) -> (element=w508:fxp<+,16,8>)
          n244 = Integer to Fixed-Point Cast(integer=u32 2) -> (fixed-point=w510:fxp<+,32,32>)  [unwired: 1 in]
          n245 = Multiply(x=w508, y=w510) -> (x*y=w505:u32)
          n246 = Subtract(x=u32 200, y=w505) -> (x-y=w512:u32)
        }
      }
    }
  }
  n247 = while {
    shift-right: [w514] -> _
    shift-left: w6 -> [w517]
    shift-right: [w515] -> _
    shift-left: w6 -> [w516]
    stop <- FALSE stop-if-true
    # "PWM Gen Motor6"
    n248 = for {
      N: 2 -> [_]
      tunnel: w517 -> [w521]
      tunnel: w516 -> [w522]
      tunnel: [w520] -> w515
      tunnel: [w519] -> w514
      i -> [w526]
      n249 = Equal To 0?(x=w526) -> (x = 0?=w523:bool)
      n250 = Select(t=w521, s=w523, f=w522) -> (s? t:f=w525:u32)
      n251 = flat-sequence {
        tunnel: w525 -> [w527]
        tunnel: [w528] -> w524
        tunnel: w523 -> [w528]
        tunnel: w524 -> [w529]
        tunnel: [w537] -> w520
        tunnel: [w530] -> w519
        frame #0 {
          n252 = call "Loop Timer7"("Count(uSec)"=w527) -> ()  [unwired: 1 out]
        }
        frame #1 {
          n253 = xnode "FPGA I/O Node"("Connector1/DIO25"=w529) -> ()  [unwired: 1 in, 1 out]
        }
        frame #2 {
          n254 = local read "PWM"() -> (w534:fxp<+,16,8>[])
          n255 = Index Array(array=w534, index=5) -> (element=w533:fxp<+,16,8>)
          n256 = Integer to Fixed-Point Cast(integer=u32 2) -> (fixed-point=w535:fxp<+,32,32>)  [unwired: 1 in]
          n257 = Multiply(x=w533, y=w535) -> (x*y=w530:u32)
          n258 = Subtract(x=u32 200, y=w530) -> (x-y=w537:u32)
        }
      }
    }
  }
  n259 = while {
    shift-right: [w539] -> _
    shift-left: w8 -> [w542]
    shift-right: [w540] -> _
    shift-left: w8 -> [w541]
    stop <- FALSE stop-if-true
    # "PWM Gen Motor4"
    n260 = for {
      N: 2 -> [_]
      tunnel: w542 -> [w546]
      tunnel: w541 -> [w547]
      tunnel: [w545] -> w540
      tunnel: [w544] -> w539
      i -> [w551]
      n261 = Equal To 0?(x=w551) -> (x = 0?=w548:bool)
      n262 = Select(t=w546, s=w548, f=w547) -> (s? t:f=w550:u32)
      n263 = flat-sequence {
        tunnel: w550 -> [w552]
        tunnel: [w553] -> w549
        tunnel: w548 -> [w553]
        tunnel: w549 -> [w554]
        tunnel: [w562] -> w545
        tunnel: [w556] -> w544
        frame #0 {
          n264 = call "Loop Timer5"("Count(uSec)"=w552) -> ()  [unwired: 1 out]
        }
        frame #1 {
          n265 = xnode "FPGA I/O Node"("Connector1/DIO15"=w554) -> ()  [unwired: 1 in, 1 out]
        }
        frame #2 {
          n266 = local read "PWM"() -> (w559:fxp<+,16,8>[])
          n267 = Index Array(array=w559, index=3) -> (element=w558:fxp<+,16,8>)
          n268 = Integer to Fixed-Point Cast(integer=u32 2) -> (fixed-point=w560:fxp<+,32,32>)  [unwired: 1 in]
          n269 = Multiply(x=w558, y=w560) -> (x*y=w556:u32)
          n270 = Subtract(x=u32 200, y=w556) -> (x-y=w562:u32)
        }
      }
    }
  }
  n271 = while {
    shift-right: [w564] -> _
    shift-left: w5 -> [w567]
    shift-right: [w565] -> _
    shift-left: w5 -> [w566]
    stop <- FALSE stop-if-true
    # "PWM Gen Motor7"
    n272 = for {
      N: 2 -> [_]
      tunnel: w567 -> [w571]
      tunnel: w566 -> [w572]
      tunnel: [w570] -> w565
      tunnel: [w569] -> w564
      i -> [w576]
      n273 = Equal To 0?(x=w576) -> (x = 0?=w573:bool)
      n274 = Select(t=w571, s=w573, f=w572) -> (s? t:f=w575:u32)
      n275 = flat-sequence {
        tunnel: w575 -> [w577]
        tunnel: [w578] -> w574
        tunnel: w573 -> [w578]
        tunnel: w574 -> [w579]
        tunnel: [w587] -> w570
        tunnel: [w580] -> w569
        frame #0 {
          n276 = call "Loop Timer8"("Count(uSec)"=w577) -> ()  [unwired: 1 out]
        }
        frame #1 {
          n277 = xnode "FPGA I/O Node"("Connector1/DIO30"=w579) -> ()  [unwired: 1 in, 1 out]
        }
        frame #2 {
          n278 = local read "PWM"() -> (w584:fxp<+,16,8>[])
          n279 = Index Array(array=w584, index=6) -> (element=w583:fxp<+,16,8>)
          n280 = Integer to Fixed-Point Cast(integer=u32 2) -> (fixed-point=w585:fxp<+,32,32>)  [unwired: 1 in]
          n281 = Multiply(x=w583, y=w585) -> (x*y=w580:u32)
          n282 = Subtract(x=u32 200, y=w580) -> (x-y=w587:u32)
        }
      }
    }
  }
  n283 = while {
    shift-right: [w589] -> _
    shift-left: w9 -> [w592]
    shift-right: [w590] -> _
    shift-left: w9 -> [w591]
    stop <- FALSE stop-if-true
    # "PWM Gen Motor3"
    n284 = for {
      N: 2 -> [_]
      tunnel: w592 -> [w596]
      tunnel: w591 -> [w597]
      tunnel: [w595] -> w590
      tunnel: [w594] -> w589
      i -> [w601]
      n285 = Equal To 0?(x=w601) -> (x = 0?=w598:bool)
      n286 = Select(t=w596, s=w598, f=w597) -> (s? t:f=w600:u32)
      n287 = flat-sequence {
        tunnel: w600 -> [w602]
        tunnel: [w603] -> w599
        tunnel: w598 -> [w603]
        tunnel: w599 -> [w604]
        tunnel: [w612] -> w595
        tunnel: [w605] -> w594
        frame #0 {
          n288 = call "Loop Timer4"("Count(uSec)"=w602) -> ()  [unwired: 1 out]
        }
        frame #1 {
          n289 = xnode "FPGA I/O Node"("Connector1/DIO10"=w604) -> ()  [unwired: 1 in, 1 out]
        }
        frame #2 {
          n290 = local read "PWM"() -> (w609:fxp<+,16,8>[])
          n291 = Index Array(array=w609, index=2) -> (element=w608:fxp<+,16,8>)
          n292 = Integer to Fixed-Point Cast(integer=u32 2) -> (fixed-point=w610:fxp<+,32,32>)  [unwired: 1 in]
          n293 = Multiply(x=w608, y=w610) -> (x*y=w605:u32)
          n294 = Subtract(x=u32 200, y=w605) -> (x-y=w612:u32)
        }
      }
    }
  }
  n295 = while {
    shift-right: [w614] -> _
    shift-left: w10 -> [w617]
    shift-right: [w615] -> _
    shift-left: w10 -> [w616]
    stop <- FALSE stop-if-true
    # "PWM Gen Motor2"
    n296 = for {
      N: 2 -> [_]
      tunnel: w617 -> [w621]
      tunnel: w616 -> [w622]
      tunnel: [w620] -> w615
      tunnel: [w619] -> w614
      i -> [w626]
      n297 = Equal To 0?(x=w626) -> (x = 0?=w623:bool)
      n298 = Select(t=w621, s=w623, f=w622) -> (s? t:f=w625:u32)
      n299 = flat-sequence {
        tunnel: w625 -> [w627]
        tunnel: [w628] -> w624
        tunnel: w623 -> [w628]
        tunnel: w624 -> [w629]
        tunnel: [w637] -> w620
        tunnel: [w630] -> w619
        frame #0 {
          n300 = call "Loop Timer3"("Count(uSec)"=w627) -> ()  [unwired: 1 out]
        }
        frame #1 {
          n301 = xnode "FPGA I/O Node"("Connector1/DIO5"=w629) -> ()  [unwired: 1 in, 1 out]
        }
        frame #2 {
          n302 = local read "PWM"() -> (w634:fxp<+,16,8>[])
          n303 = Index Array(array=w634, index=1) -> (element=w633:fxp<+,16,8>)
          n304 = Integer to Fixed-Point Cast(integer=u32 2) -> (fixed-point=w635:fxp<+,32,32>)  [unwired: 1 in]
          n305 = Multiply(x=w633, y=w635) -> (x*y=w630:u32)
          n306 = Subtract(x=u32 200, y=w630) -> (x-y=w637:u32)
        }
      }
    }
  }
  n307 = while {
    shift-right: [w639] -> _
    shift-left: w4 -> [w642]
    shift-right: [w640] -> _
    shift-left: w4 -> [w641]
    stop <- FALSE stop-if-true
    # "PWM Gen Motor1"
    n308 = for {
      N: 2 -> [_]
      tunnel: w642 -> [w646]
      tunnel: w641 -> [w647]
      tunnel: [w645] -> w640
      tunnel: [w644] -> w639
      i -> [w651]
      n309 = Equal To 0?(x=w651) -> (x = 0?=w648:bool)
      n310 = Select(t=w646, s=w648, f=w647) -> (s? t:f=w650:u32)
      n311 = flat-sequence {
        tunnel: w650 -> [w652]
        tunnel: [w653] -> w649
        tunnel: w648 -> [w653]
        tunnel: w649 -> [w654]
        tunnel: [w662] -> w645
        tunnel: [w655] -> w644
        frame #0 {
          n312 = call "Loop Timer2"("Count(uSec)"=w652) -> ()  [unwired: 1 out]
        }
        frame #1 {
          n313 = xnode "FPGA I/O Node"("Connector1/DIO0"=w654) -> ()  [unwired: 1 in, 1 out]
        }
        frame #2 {
          n314 = local read "PWM"() -> (w659:fxp<+,16,8>[])
          n315 = Index Array(array=w659, index=0) -> (element=w658:fxp<+,16,8>)
          n316 = Integer to Fixed-Point Cast(integer=u32 2) -> (fixed-point=w660:fxp<+,32,32>)  [unwired: 1 in]
          n317 = Multiply(x=w658, y=w660) -> (x*y=w655:u32)
          n318 = Subtract(x=u32 200, y=w655) -> (x-y=w662:u32)
        }
      }
    }
  }
  n319 = while {
    stop <- FALSE stop-if-true
    n320 = flat-sequence {
      frame #0 {
        n321 = call "Loop Timer10"("Count(uSec)"=u32 200) -> ()  [unwired: 1 out]
      }
      frame #1 {
        n322 = local read "AmpCmd"() -> (w678:sgl[])
        n323 = Divide(x=w678, y=i16 10) -> (x/y=w676:sgl[])
        n324 = Scale By Power Of 2(n=i16 15, x=w676) -> (x*2^n=w674:sgl[])
        n325 = To Word Integer(number=w674) -> (16bit integer=w673:i16[])
        n326 = Index Array(array=w673) -> (element #1=w672:i16, element #2=w671:i16, element #3=w670:i16, element #4=w669:i16, element #5=w668:i16, element #6=w667:i16, element #7=w666:i16, element #8=w665:i16)  [unwired: 8 in]
        n327 = xnode "FPGA I/O Node"("Connector0/AO0"=w672, "Connector0/AO1"=w671, "Connector0/AO2"=w670, "Connector0/AO3"=w669, "Connector0/AO4"=w668, "Connector0/AO5"=w667, "Connector0/AO6"=w666, "Connector0/AO7"=w665) -> ()  [unwired: 8 in, 8 out]
      }
    }
  }
  n328 = while {
    stop <- FALSE stop-if-true
    n329 = stacked-sequence {
      frame #0 {
        n330 = global read "GVEncoder.vi" "EncdCnt 8"() -> (w680:fxp<+/-,32,32>)
        n331 = global read "GVEncoder.vi" "EncdPos 1"() -> (w694:fxp<+/-,32,32>)
        n332 = global read "GVEncoder.vi" "EncdPos 2"() -> (w693:fxp<+/-,32,32>)
        n333 = global read "GVEncoder.vi" "EncdPos 3"() -> (w692:fxp<+/-,32,32>)
        n334 = global read "GVEncoder.vi" "EncdPos 4"() -> (w686:fxp<+/-,32,32>)
        n335 = global read "GVEncoder.vi" "EncdPos 5"() -> (w685:fxp<+/-,32,32>)
        n336 = global read "GVEncoder.vi" "EncdPos 6"() -> (w684:fxp<+/-,32,32>)
        n337 = global read "GVEncoder.vi" "EncdPos 7"() -> (w683:fxp<+/-,32,32>)
        n338 = xnode ("High Throughput Multiply")("x"="EncoderCount", "y"=fxp<+,4,4> 4.0) -> ("x*y"=w688:fxp<+,16,16>)
        n339 = xnode "High Throughput Divide"("x"="2pi", "y"=w688) -> ("x/y"=w681:fxp<+/-,32,4>)
        n340 = Build Array(w694, w693, w692, w686, w685, w684, w683, w680) -> (w682:fxp<+/-,32,32>[])
        n341 = Multiply(x=w682, y=w681) -> (x*y=w690:fxp<+/-,32,16>[])
        n342 = To Single Precision Float(number=w690) -> (single precision float=→"EncdAngle":sgl[])
      }
      frame #1 {
        n343 = call "Loop Timer"("Count(uSec)"=u32 1) -> ()  [unwired: 1 out]
      }
    }
  }
